vi "Read Step.vi"(8 "error in (no error)":errorcluster, 11 "Voltage with Increment in":refnum<class "Voltage with Step.lvclass">) -> (0 "error out":errorcluster, 2 "Step":dbl=inf min=inf step=0.001, 3 "Voltage with Increment out":refnum<class "Voltage with Step.lvclass">)   [LabVIEW 2023, in "HAF.lvlib" / "Voltage with Step.lvclass"]
uses:
  Voltage with Step.lvclass
  Voltage with Step.lvclass/Voltage with Step.ctl
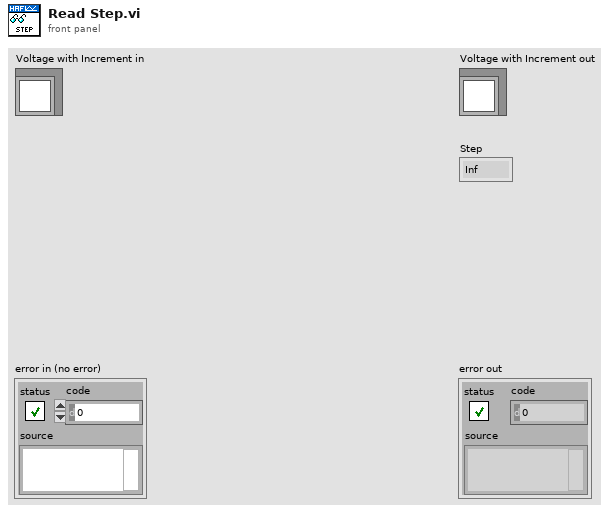
[diagram p1: front panel]
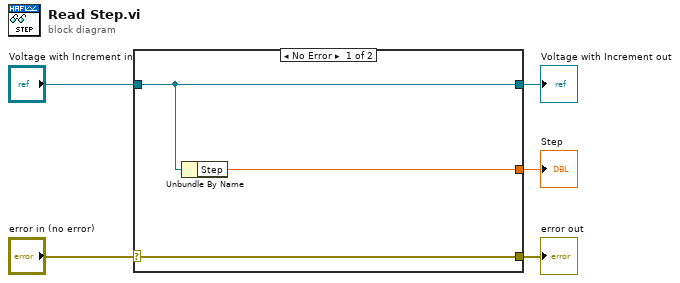
[diagram p0: block diagram]
diagram:
  n1 = case shown="No Error" "error in (no error)" {
    selector: "error in (no error)" -> [w8 w9]
    tunnel: [w8 w9] -> w4
    tunnel: [w7 w10] -> w2
    tunnel: "Voltage with Increment in" -> [w7 w10]
    tunnel: [w6 _] -> w1
    frame No Error {
      n2 = Unbundle By Name(w7) -> ("Step"=w6:dbl)
    }
    frame Error {
    }
  }
  "error out" <- w4
  "Voltage with Increment out" <- w2
  "Step" <- w1
